vi "DAQ - Check and Reserve.vi"(8 "error in":errorcluster, 11 "Device":tag) -> (0 "error out":errorcluster, 3 "Modules":tag[](array[tag]))   [LabVIEW 2021]
doc: "Given a device name, this VI will attempt to contact the DAQ, and return an array of DAQ modules if it succeeds. If it fails, it will attempt to reserve the device. If this fails to reserve, it will then return an error."
uses:
  <resource>/objmgr/daqmx.rc
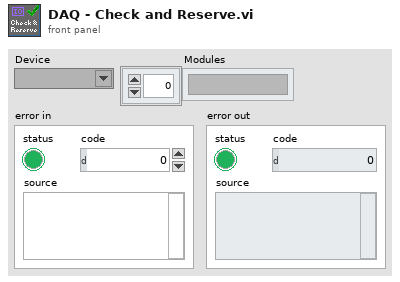
[diagram p1: front panel]
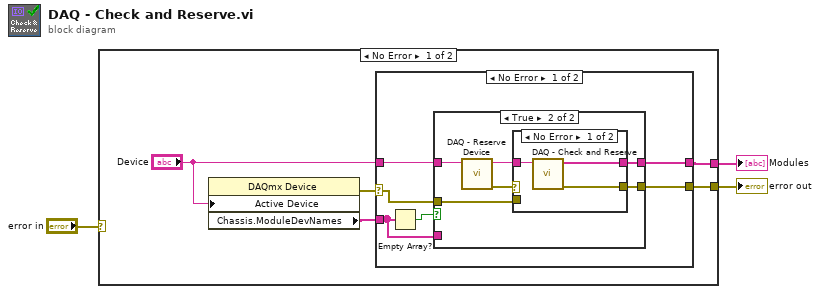
[diagram p0: block diagram]
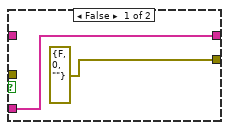
[diagram p2: hidden frame]
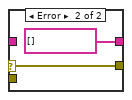
[diagram p3: hidden frame]
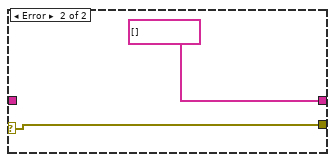
[diagram p4: hidden frame]
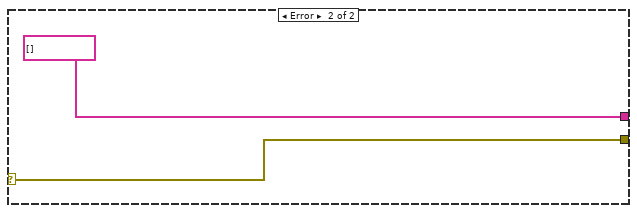
[diagram p5: hidden frame]
diagram:
  n1 = case shown="No Error" "error in" {
    selector: "error in" -> [_ w30]
    tunnel: [w5 tag[] [] ("Modules")] -> w2
    tunnel: [w4 w30] -> w1
    frame No Error {
      n2 = property class="DAQmx Device"("Active Device"="Device") -> (error out=w8:errorcluster, "Chassis.ModuleDevNames"=w7:tag[])  [unwired: 2 in, 1 out]
      n3 = case shown="No Error" w8 {
        selector: w8 -> [w12 w29]
        tunnel: w7 -> [w9 _]
        tunnel: "Device" -> [w14 _]
        tunnel: [w13 w29] -> w4
        tunnel: [w11 tag[] [] ("Modules")] -> w5
        frame No Error {
          n4 = Empty Array?(array=w9) -> (empty?=w10:bool)
          n5 = case shown="True" w10 {
            tunnel: w14 -> [_ w19]
            tunnel: [errorcluster {"status"=FALSE, "code"=0, "source"=""} ("error IO") w22] -> w13
            tunnel: w12 -> [_ w21]
            tunnel: [w16 w20] -> w11
            tunnel: w9 -> [w16 _]
            frame False {
            }
            frame True {
              n6 = call "DAQ - Reserve Device.vi"("device in"=w19) -> ("error out"=w17:errorcluster, "device out"=w18:tag)  [unwired: 9 in]
              n7 = case shown="No Error" w17 {
                selector: w17 -> [_ w26]
                tunnel: w18 -> [w25 _]
                tunnel: [w24 w26] -> w22
                tunnel: w21 -> [_ _]
                tunnel: [w23 tag[] [] ("Modules")] -> w20
                frame No Error {
                  n8 = call "DAQ - Check and Reserve.vi"("Device"=w25) -> ("error out"=w24:errorcluster, "Modules"=w23:tag[])  [unwired: 9 in]
                }
                frame Error {
                }
              }
            }
          }
        }
        frame Error {
        }
      }
    }
    frame Error {
    }
  }
  "error out" <- w1
  "Modules" <- w2
